vi "setUp.vi"(8 "error in (no error)":errorcluster, 11 "reference in":refnum<class "Max Nr of Scalar Channels.lvclass">) -> (0 "error out":errorcluster, 3 "reference out":refnum<class "Max Nr of Scalar Channels.lvclass">)   [LabVIEW 2019, in "Max Nr of Scalar Channels.lvclass"]
doc: "setUp runs prior to the test method during test execution. Use this method to initialize any object data required by your tests."
uses:
  Max Nr of Scalar Channels.lvclass
  C:/Program Files (x86)/National Instruments/LabVIEW 2019/vi.lib/addons/_JKI Toolkits/VI Tester/TestCase.llb/TestCase.lvclass
  Max Nr of Scalar Channels.lvclass/Max Nr of Scalar Channels.ctl
  FPGA Addon Test Class/FPGA Addon Test Class.lvclass
  C:/Dev/niveristand-fpga-addon-custom-device/Source/Tests/FPGA Addon Test Class/FPGA Addon Test Class.lvclass
  C:/Dev/niveristand-custom-device-testing-tools/VeriStandTestCase/VeriStandTestCase.lvclass
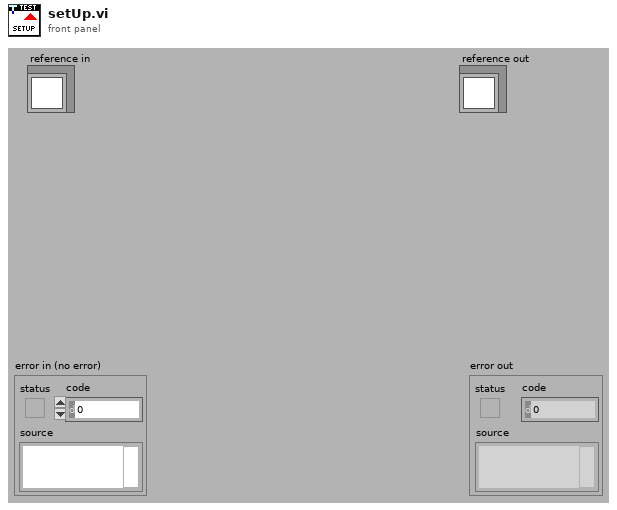
[diagram p1: front panel]
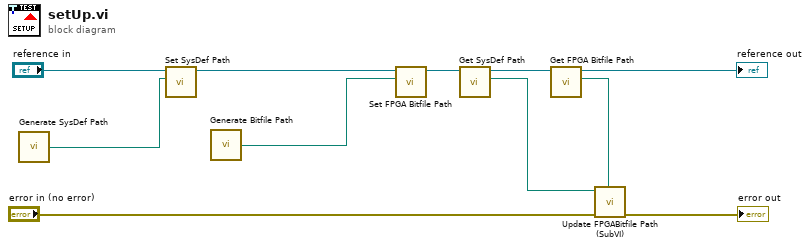
[diagram p0: block diagram]
diagram:
  n1 = call "Generate SysDef Path.vi"() -> ("System Definition path"=w7:path)
  n2 = call "Set SysDef Path.vi"("SysDef Path"=w7, "Scalar Channels Testing in"="reference in") -> ("Scalar Channels Testing out"=w11:refnum<class "Max Nr of Scalar Channels.lvclass">)  [unwired: 9 in]
  n3 = call "Generate Bitfile Path.vi"() -> ("System Definition path"=w6:path)
  n4 = call "Set FPGA Bitfile Path.vi"("FPGA Bitfile Path"=w6, "Scalar Channels Testing in"=w11) -> ("Scalar Channels Testing out"=w10:refnum<class "Max Nr of Scalar Channels.lvclass">)  [unwired: 9 in]
  n5 = call "Get SysDef Path.vi"("Scalar Channels Testing in"=w10) -> ("SysDef Path"=w4:path, "Scalar Channels Testing out"=w9:refnum<class "Max Nr of Scalar Channels.lvclass">)  [unwired: 9 in]
  n6 = call "Get FPGA Bitfile Path.vi"("Scalar Channels Testing in"=w9) -> ("FPGA Bitfile Path"=w5:path, "Scalar Channels Testing out"=→"reference out":refnum<class "Max Nr of Scalar Channels.lvclass">)  [unwired: 9 in]
  n7 = call "Update FPGABitfile Path (SubVI).vi"("Bitfile Path"=w5, "error in (no error)"="error in (no error)", "System Definition path in"=w4) -> ("error out"=→"error out":errorcluster)  [unwired: 7 in, 1 out]
